vi "DICTIONARY_subdictionaryExample.vi"() -> ()   [LabVIEW 2016]
uses:
  <userlib>/_OpenG.lib/dictionary/dictionary.llb/Dictionary Object RefNum__ogtk.ctl
  <userlib>/_OpenG.lib/dictionary/dictionary.llb/Dictionary Object RefNum - Enum__ogtk.ctl
  <userlib>/_OpenG.lib/dictionary/dictionary.llb/Dictionary Update (by scalar value)__ogtk.vi
panel:
  out "subvalue":variant
  out "value":variant
  out "dictionary out":T1
  out "Dictionary Items":cluster{"key":variant, "value":variant}[](array[cluster])
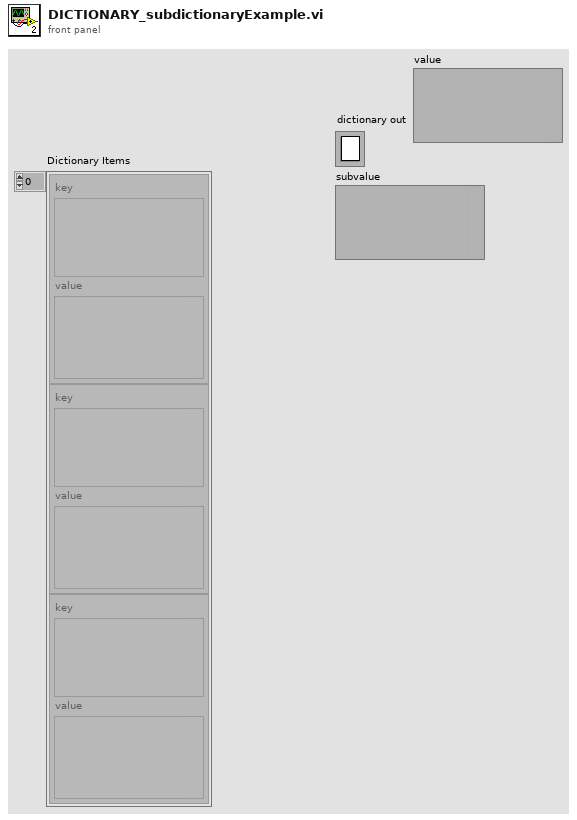
[diagram p1: front panel]
types:
  T1 = typedef "Dictionary Object RefNum__ogtk.ctl" = refnum<k1>
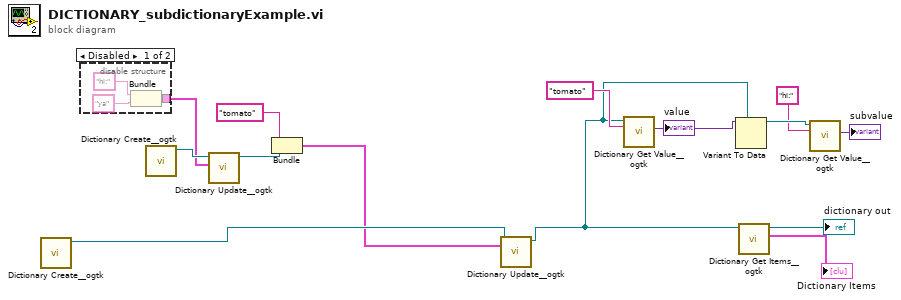
[diagram p0: block diagram]
diagram:
  n1 = call <userlib>:"Dictionary Create__ogtk.vi"() -> ("dictionary out"=w12:T1)  [unwired: 10 in, 1 out]
  n2 = disable-structure shown="Disabled" {
    disable-tunnel: [w15 _] -> w5
    frame Disabled {
      n3 = Bundle("hi:", "ya") -> (w15:cluster{string, string})  [unwired: 1 in]
    }
    frame Enabled {
    }
  }
  n4 = call <userlib>:"Dictionary Create__ogtk.vi"() -> ("dictionary out"=w6:T1)  [unwired: 10 in, 1 out]
  n5 = call-poly <userlib>:"Dictionary Update__ogtk.vi"("key-value"=w5, "dictionary"=w6) -> ("dictionary out"=w4:T1)  [unwired: 7 in, 2 out]
  n6 = Bundle("tomato", "dictionary out"=w4) -> (w10:cluster{string, "dictionary out":T1})  [unwired: 1 in]
  n7 = call-poly <userlib>:"Dictionary Update__ogtk.vi"("key-value"=w10, "dictionary"=w12) -> ("dictionary out"=w7:T1)  [unwired: 7 in, 2 out]
  n8 = call <userlib>:"Dictionary Get Value__ogtk.vi"("key"="tomato", "dictionary"=w7) -> ("value"=w8:variant)  [unwired: 6 in, 3 out]
  "value" <- w8
  n9 = Variant To Data(type=w7, Variant=w8) -> (data=w3:T1)  [unwired: 1 in, 1 out]
  n10 = call <userlib>:"Dictionary Get Items__ogtk.vi"("dictionary"=w7) -> ("items"=→"Dictionary Items":cluster{"key":variant, "value":variant}[], "dictionary out"=→"dictionary out":T1)  [unwired: 8 in, 1 out]
  n11 = call <userlib>:"Dictionary Get Value__ogtk.vi"("key"="hi:", "dictionary"=w3) -> ("value"=→"subvalue":variant)  [unwired: 6 in, 3 out]
